vi "RD Analog Out Node Function Set.vi"(7 "func":T1(ring), 8 "error in (no error)":errorcluster caption="错误输入（无错误）", 9 "node":i32, 10 "ch":i32, 11 "handle":u64) -> (0 "error out":errorcluster caption="错误输出", 2 "function return":i32, 3 "handle out":u64)   [LabVIEW 2018, in "InstrumentsPlayground.lvlib"]
doc: "CLIFFAPI int CliffAnalogOutNodeFunctionSet(FT_HANDLE handle, int ch, CLIFFAnalogOutNode node, CLIFFFUNC func);\nch: 0 ch1; 1 ch2;\nnode: Carrier = 0;FM = 1;AM = 2;\nfunc:\nDC = 0;\nSine = 1;\nSquare = 2;\nTriangle = 3;\nRampUp = 4;\nRampDown = 5;\nNoise = 6;\nPulse = 7;\nTrapezium= 8;\nSinePower= 9;\nCustom = 30;\nPlay = 31;"
uses:
  InstrumentsPlayground.lvlib
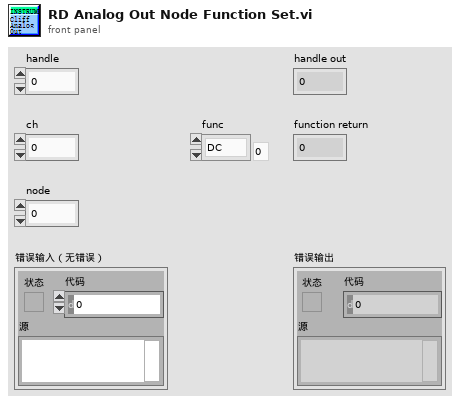
[diagram p1: front panel]
types:
  T1 = enum8{"DC", "Sine", "Square", "Triangle", "RampUp", "RampDown", "Noise", "Pulse", "Trapezium", "SinePower", "Custom", "Play"}
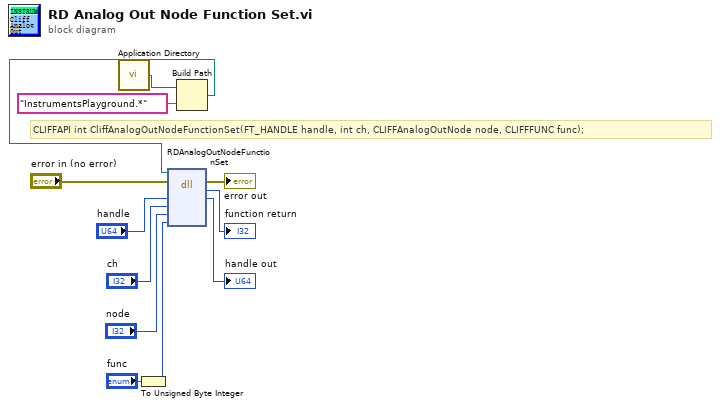
[diagram p0: block diagram]
diagram:
  # "CLIFFAPI int CliffAnalogOutNodeFunctionSet(FT_HANDLE handle, int ch, CLIFFAnalogOutNode node, CLIFFFUNC func);"
  n1 = call <vilib>:"Application Directory.vi"() -> ("Application Directory"=w3:path)
  n2 = To Unsigned Byte Integer(number="func") -> (unsigned 8bit integer=w1:u8)
  n3 = Build Path(base path=w3, name or relative path="InstrumentsPlayground.*" ("名称或相对路径")) -> (appended path=w2:path)
  n4 = dll-call lib="E:/work/YZCourse_Xtext/Cliff/API/LabVIEW lib/InstrumentsPlayground.*" fn="RDAnalogOutNodeFunctionSet"(path in=w2, error in="error in (no error)", "handle"="handle", "ch"="ch", "node"="node", "func"=w1) -> (error out=→"error out":errorcluster, "返回类型"=→"function return":i32, "handle"=→"handle out":u64)  [unwired: 4 in, 1 out]
